vi "Write Parser.vi"(8 "Error In":errorcluster, 10 "Parser":refnum<class "Parser.lvclass">, 11 "Compiler In":refnum<class "Compiler.lvclass">) -> (0 "Error Out":errorcluster, 3 "Compiler Out":refnum<class "Compiler.lvclass">)   [LabVIEW 2018, in "Toolkit.lvlib" / "Compiler.lvclass"]
uses:
  Compiler.lvclass
  Parser/Parser.lvclass
  Compiler.lvclass/Compiler.ctl
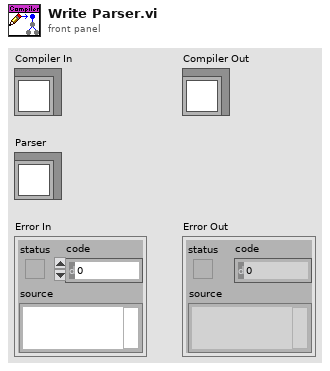
[diagram p1: front panel]
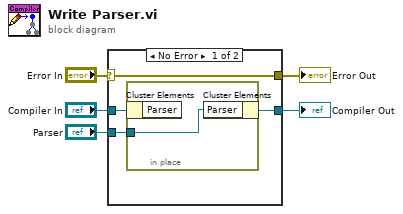
[diagram p0: block diagram]
diagram:
  n1 = case shown="No Error" "Error In" {
    selector: "Error In" -> [w9 w11]
    tunnel: [w9 w11] -> w4
    tunnel: [w6 w12] -> w2
    tunnel: "Compiler In" -> [w8 w12]
    tunnel: "Parser" -> [w7 _]
    frame No Error {
      n2 = in-place {
        in-place-border: w7 -> [w10]
        n3 = in-place-cluster #1(w8) -> ()  [unwired: 1 out]
        n4 = in-place-cluster #1("Parser"=w10) -> (w6:refnum<class "Compiler.lvclass">)
      }
    }
    frame Error {
    }
  }
  "Error Out" <- w4
  "Compiler Out" <- w2
